vi "CRYDataView Add Panel.vi"(6 "DataView Index":i32, 7 "panel_index":i32, 8 "Selected Panel Idx":i32, 9 "SAdd_Pos":string, 10 "spliter array":refnum<vi>[](array[refnum]), 11 "SubPanel array":refnum<vi>[](array[refnum])) -> (1 "Panel Ref":refnum<vi>, 2 "bResult":bool, 3 "panel_index_out":i32)   [LabVIEW 2013]
uses:
  Control/SplitterBar.ctl
  CRYNew View Global.vi
panel:
  in  "V or H":i32
  in  "cur_position":i32
  in  "parent_spliteridx":i32
  in  "new_add_position":i32
  in  "panel_left":i32
  in  "panel_top":i32
  in  "panel_right":i32
  in  "panel_btm":i32
  in  "cur_panel_top":i32
  in  "cur_panel_left":i32
  in  "cur_panel_hei":i32
  in  "cur_panel_wid":i32
  in  "spliter_index":i32
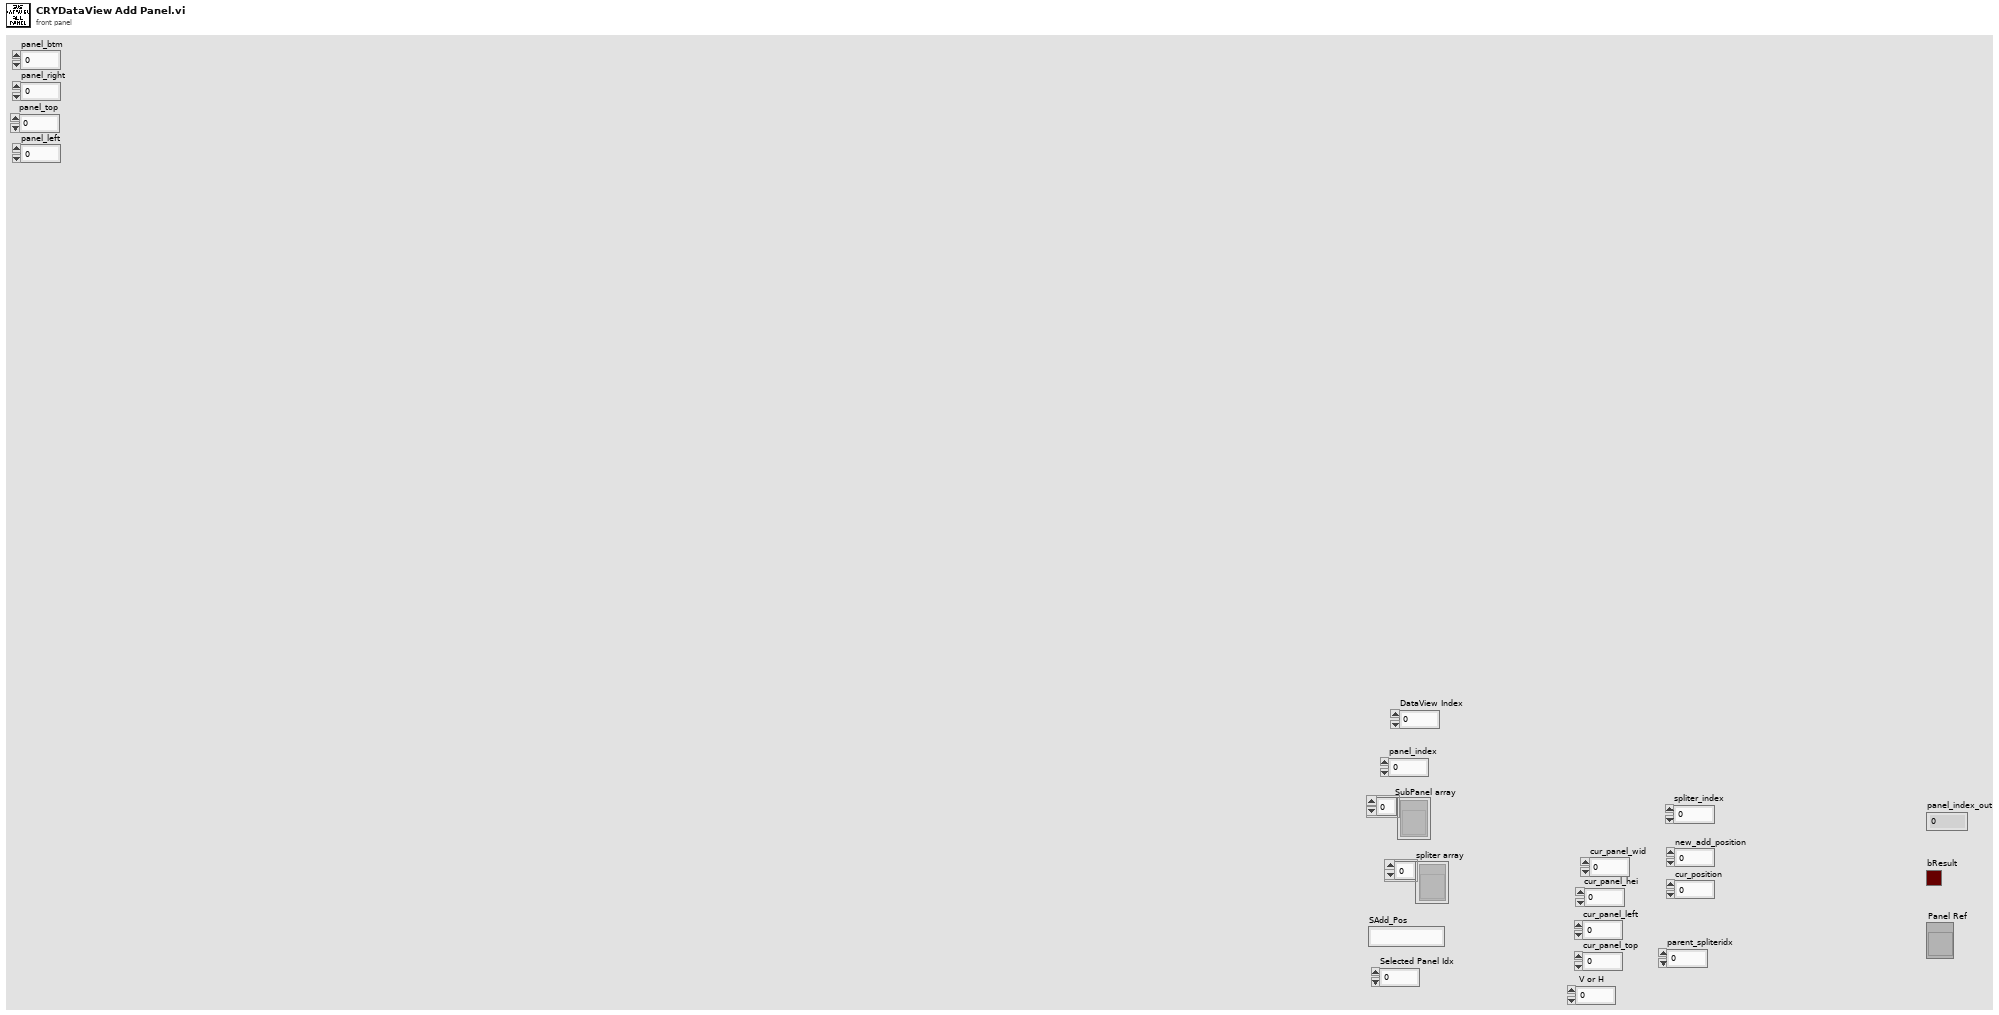
[diagram p1: front panel]
types:
  T1 = typedef "Graph Main Info Cluster.ctl" = cluster{"Selected_BarIdx":i32, "Selected_PanelIdx":i32, "Graph Main VIRef":refnum<vi>, "ToolBarClick":bool, "Spliter Ref Array":refnum<vi>[], "Panel Ref Array":refnum<vi>[], "Spliter_matrix":i32[][], "Panel_matrix":i32[][], "child_spliterIdx_matrix":i32[][], "split_pos_matrix":i32[][], "Title State":bool, "sQueueName":string, "Frame nID":i32, "Graph VIRef Array":cluster{"Graph VIRef":refnum<vi>, "Panel Idx":i32, "Frame VIRef":refnum<vi>, "Icon Ring":i32, "Graph Type":string}[], "View Type":string}
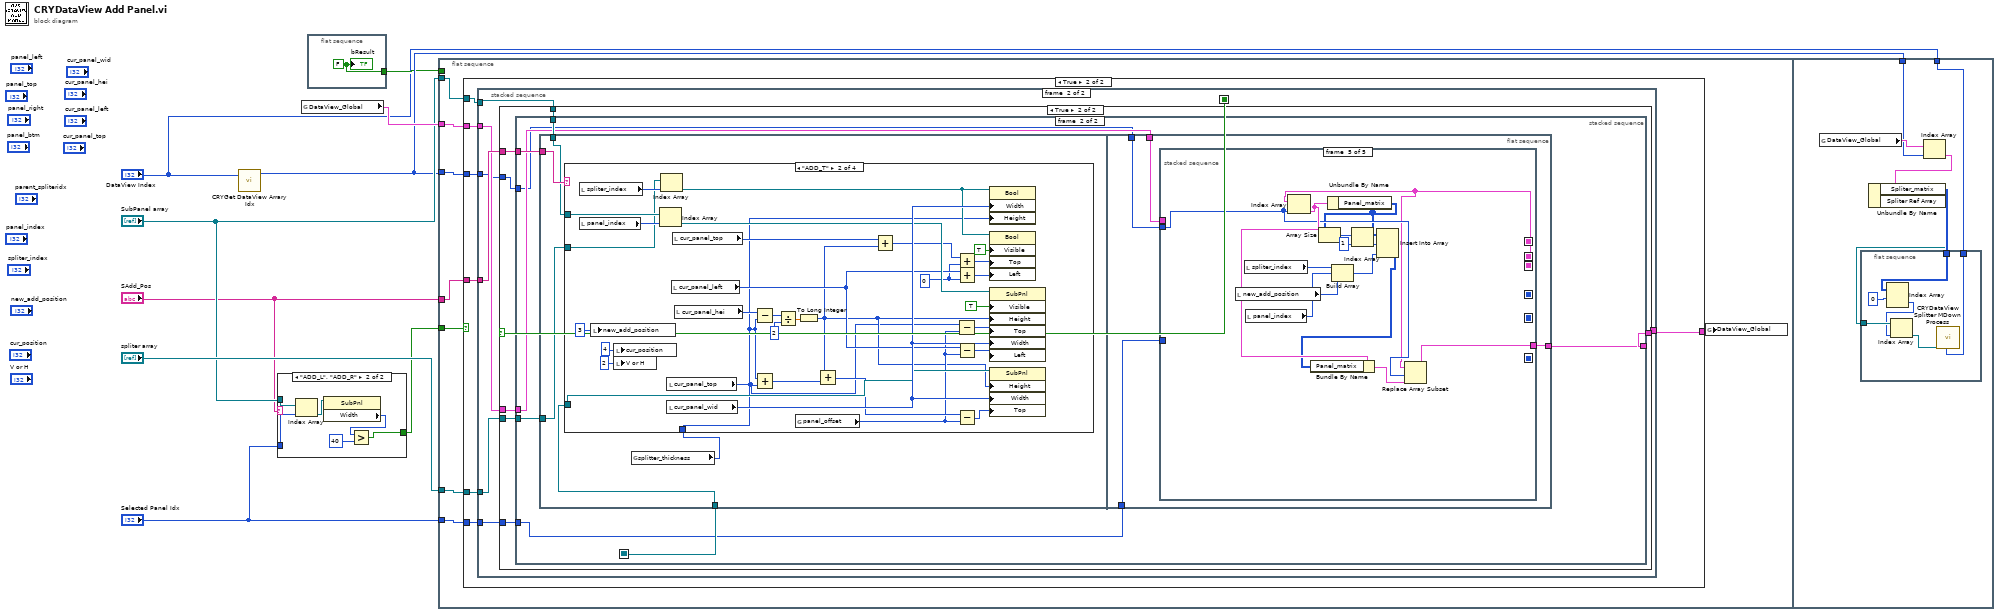
[diagram p0: block diagram]
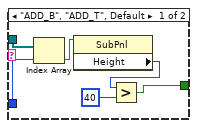
[diagram p2: hidden frame]
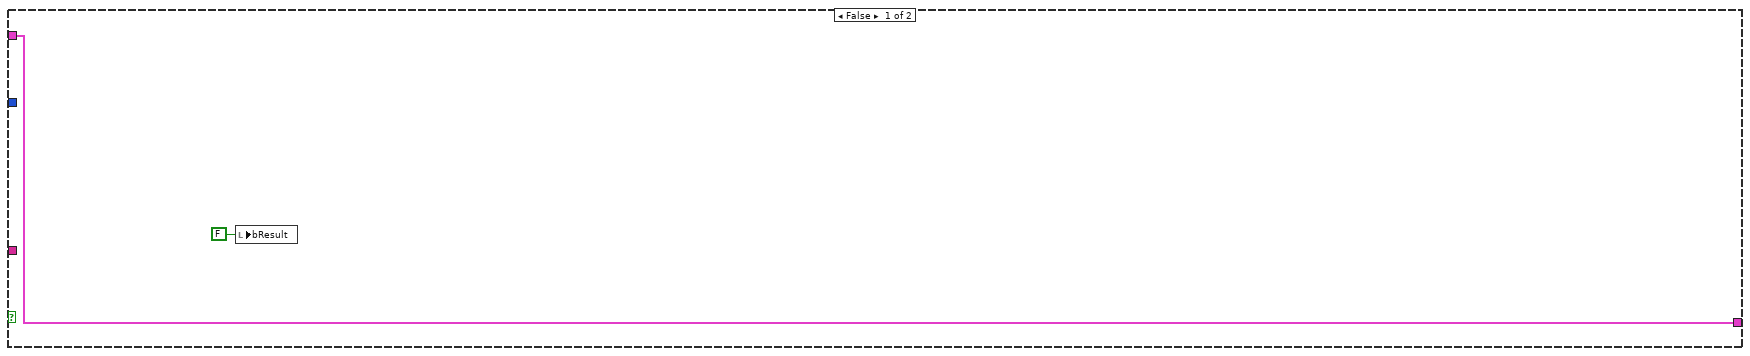
[diagram p3: hidden frame]
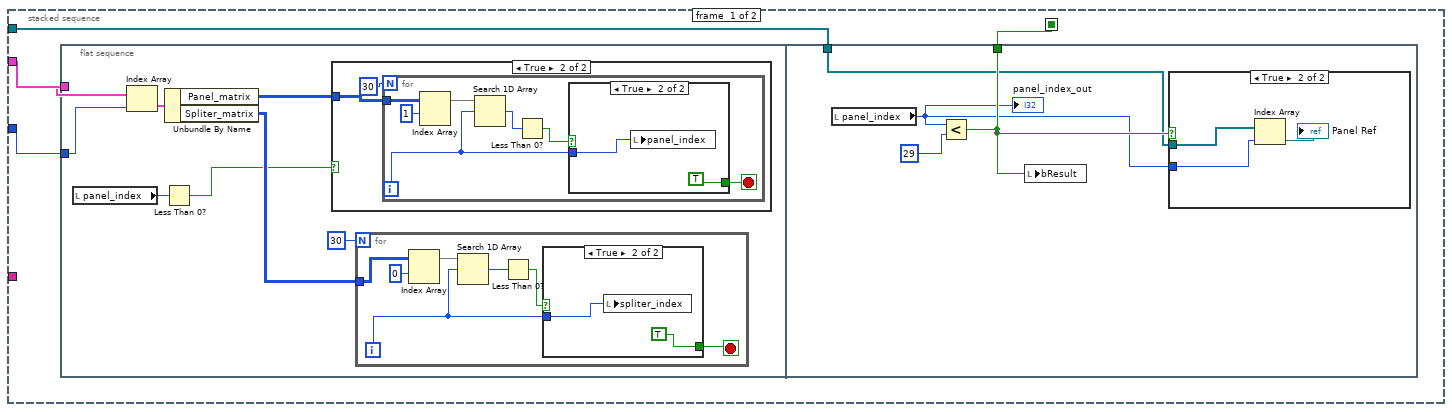
[diagram p4: hidden frame]
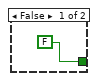
[diagram p6: hidden frame]
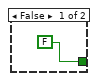
[diagram p7: hidden frame]
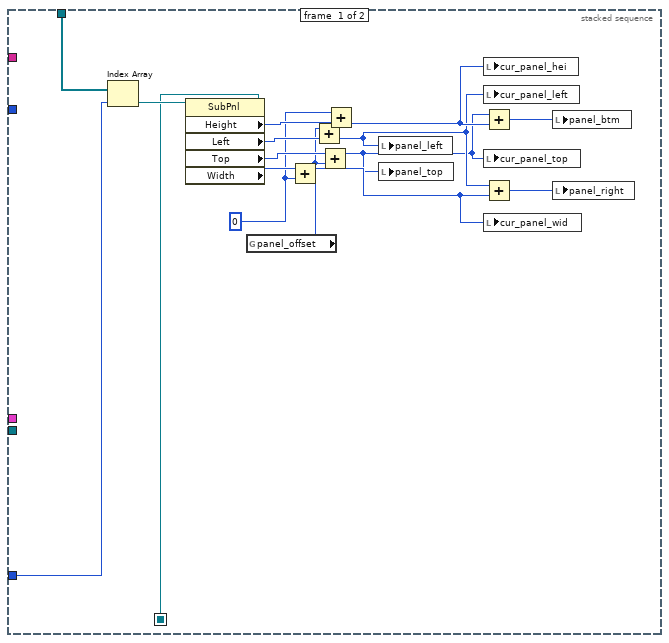
[diagram p10: hidden frame]
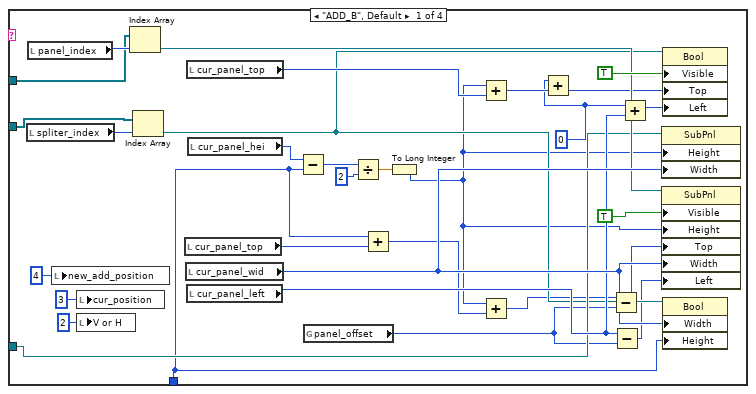
[diagram p11: hidden frame]
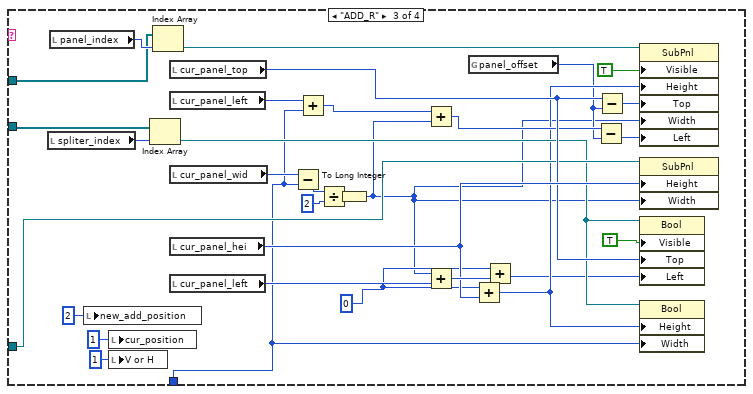
[diagram p12: hidden frame]
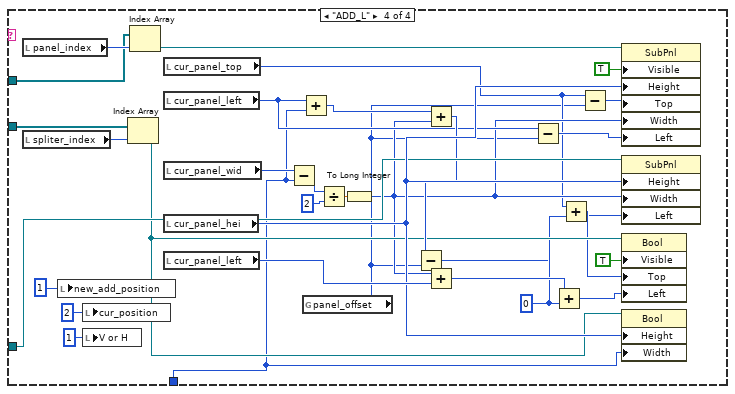
[diagram p13: hidden frame]
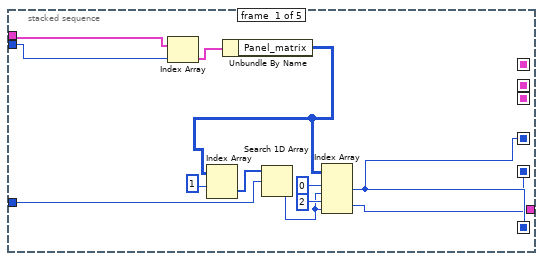
[diagram p14: hidden frame]
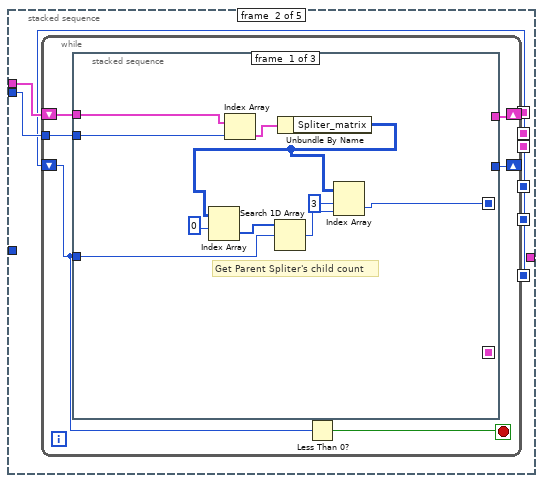
[diagram p15: hidden frame]
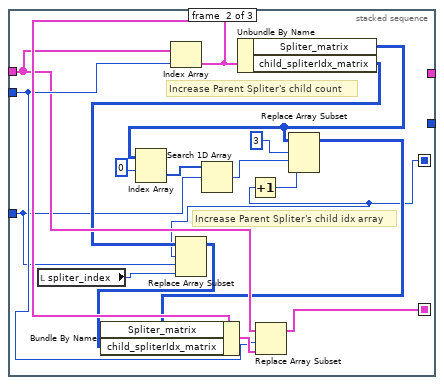
[diagram p16: hidden frame]
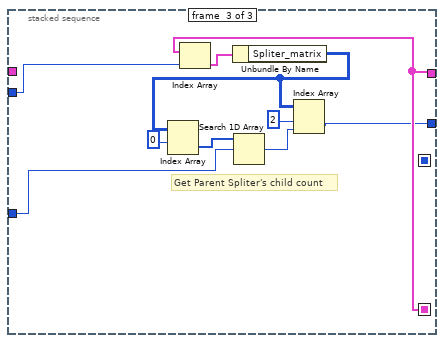
[diagram p17: hidden frame]
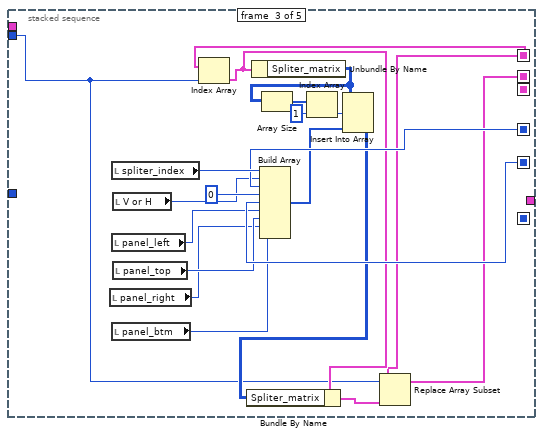
[diagram p18: hidden frame]
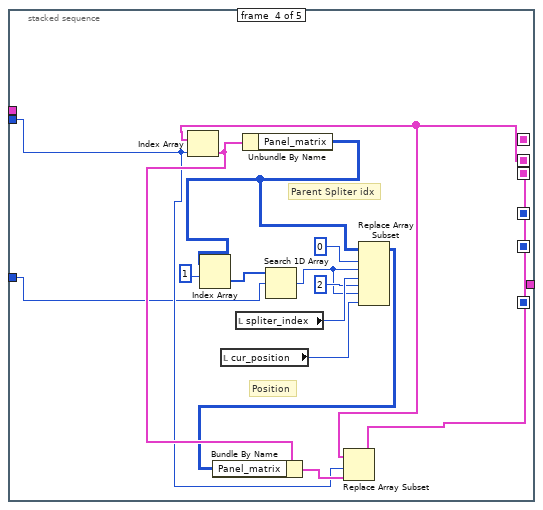
[diagram p19: hidden frame]
diagram:
  n1 = call "CRYGet DataView Arrary Idx.vi"("DataView Idx In"="DataView Index") -> ("DataView Arrary Idx out"=w3:i32)  [unwired: 10 in]
  n2 = case shown="\"ADD_L\", \"ADD_R\"" "SAdd_Pos" {
    tunnel: "Selected Panel Idx" -> [w15 w21]
    tunnel: "SubPanel array" -> [w14 w20]
    tunnel: [w10 w16] -> w4
    frame "ADD_B", "ADD_T", Default {
      n3 = Index Array(array=w14, index=w15) -> (element=w13:refnum<vi>)
      n4 = property class="SubPnl"(reference=w13) -> ("Height"=w12:u32)  [unwired: 1 in, 2 out]
      n5 = Greater?(x=w12, y=u32 40) -> (0:w10:bool)
    }
    frame "ADD_L", "ADD_R" {
      n6 = Index Array(array=w20, index=w21) -> (element=w19:refnum<vi>)
      n7 = property class="SubPnl"(reference=w19) -> ("Width"=w18:u32)  [unwired: 1 in, 2 out]
      n8 = Greater?(x=w18, y=u32 40) -> (0:w16:bool)
    }
  }
  n9 = global read "CRYNew View Global.vi" "DataView_Global"() -> (w9:T1[])
  n10 = flat-sequence {
    tunnel: [w22] -> w2
    frame #0 {
      w22 = FALSE ("bResult")
      "bResult" <- w22
    }
  }
  n11 = flat-sequence {
    tunnel: "SubPanel array" -> [w30]
    tunnel: "spliter array" -> [w29]
    tunnel: "SAdd_Pos" -> [w28]
    tunnel: w9 -> [w27]
    tunnel: w3 -> [w26]
    tunnel: "Selected Panel Idx" -> [w24]
    tunnel: w4 -> [w23]
    tunnel: w2 -> [_]
    tunnel: w3 -> [w365]
    tunnel: "DataView Index" -> [w364]
    frame #0 {
      n12 = case shown="True" w23 {
        tunnel: w30 -> [_ w39]
        tunnel: w29 -> [_ w38]
        tunnel: w28 -> [_ w37]
        tunnel: w27 -> [w32 w36]
        tunnel: w26 -> [_ w35]
        tunnel: [w32 w34] -> w25
        tunnel: w24 -> [_ w33]
        frame False {
          n13 = local write "bResult"(FALSE ("bResult")) -> ()
        }
        frame True {
          n14 = stacked-sequence {
            seq-local: [w40 _] -> [_ w82]
            tunnel: w36 -> [w43 w85]
            tunnel: w35 -> [w42 w84]
            tunnel: w39 -> [w41 w87]
            tunnel: w37 -> [_ w88]
            tunnel: w38 -> [_ w86]
            tunnel: [_ w83] -> w34
            tunnel: w33 -> [_ w81]
            frame #0 {
              n15 = flat-sequence {
                tunnel: w43 -> [w51]
                tunnel: w42 -> [w50]
                tunnel: w41 -> [w75]
                tunnel: [w76] -> w40
                frame #0 {
                  n16 = local read "panel_index"() -> (w49:i32)
                  n17 = Index Array(array=w51, index=w50) -> (element=w47:T1)
                  n18 = Less Than 0?(x=w49) -> (x < 0?=w44:bool)
                  n19 = Unbundle By Name(w47) -> ("Panel_matrix"=w46:i32[][], "Spliter_matrix"=w45:i32[][])
                  n20 = case shown="True" w44 {
                    tunnel: w46 -> [_ w52]
                    frame False {
                    }
                    frame True {
                      n21 = for {
                        N: 30 -> [_]
                        tunnel: w52 -> [w54]
                        i -> [w56]
                        stop <- w55 stop-if-true
                        n22 = Index Array(array=w54, index (row)=1) -> (element=w59:i32[])  [unwired: 1 in]
                        n23 = Search 1D Array(1D array=w59, element=w56) -> (index of element=w58:i32)  [unwired: 1 in]
                        n24 = Less Than 0?(x=w58) -> (x < 0?=w57:bool)
                        n25 = case shown="True" w57 {
                          tunnel: w56 -> [_ w63]
                          tunnel: [FALSE TRUE] -> w55
                          frame False {
                          }
                          frame True {
                            n26 = local write "panel_index"(w63) -> ()
                          }
                        }
                      }
                    }
                  }
                  n27 = for {
                    N: 30 -> [_]
                    tunnel: w45 -> [w64]
                    i -> [w66]
                    stop <- w65 stop-if-true
                    n28 = Index Array(array=w64, index (row)=0) -> (element=w69:i32[])  [unwired: 1 in]
                    n29 = Search 1D Array(1D array=w69, element=w66) -> (index of element=w68:i32)  [unwired: 1 in]
                    n30 = Less Than 0?(x=w68) -> (x < 0?=w67:bool)
                    n31 = case shown="True" w67 {
                      tunnel: w66 -> [_ w73]
                      tunnel: [FALSE TRUE] -> w65
                      frame False {
                      }
                      frame True {
                        n32 = local write "spliter_index"(w73) -> ()
                      }
                    }
                  }
                }
                frame #1 {
                  n33 = local read "panel_index"() -> (w74:i32)
                  "panel_index_out" <- w74
                  n34 = Less?(x=w74, y=29) -> (x < y?=w76:bool)
                  n35 = local write "bResult"(w76) -> ()
                  n36 = case shown="True" w76 {
                    tunnel: w75 -> [_ w80]
                    tunnel: w74 -> [_ w79]
                    frame False {
                    }
                    frame True {
                      n37 = Index Array(array=w80, index=w79) -> (element=→"Panel Ref":refnum<vi>)
                    }
                  }
                }
              }
            }
            frame #1 {
              n38 = case shown="True" w82 {
                tunnel: w88 -> [_ w96]
                tunnel: w87 -> [_ w95]
                tunnel: w86 -> [_ w94]
                tunnel: w85 -> [w89 w93]
                tunnel: w84 -> [_ w92]
                tunnel: [w89 w91] -> w83
                tunnel: w81 -> [_ w90]
                frame False {
                }
                frame True {
                  n39 = stacked-sequence {
                    seq-local: [w104 _] -> [_ w117]
                    tunnel: w96 -> [_ w120]
                    tunnel: w95 -> [w105 w119]
                    tunnel: w94 -> [_ w118]
                    tunnel: w93 -> [_ w116]
                    tunnel: w92 -> [_ w115]
                    tunnel: [_ w114] -> w91
                    tunnel: w90 -> [w103 w113]
                    frame #0 {
                      w100 = 0
                      n40 = Index Array(array=w105, index=w103) -> (element=w106:refnum<vi>)
                      n41 = property class="SubPnl"(reference=w106) -> (reference out=w104:refnum<vi>, "Height"=w111:u32, "Left"=w107:i32, "Top"=w110:i32, "Width"=w109:u32)  [unwired: 1 in, 1 out]
                      n42 = global read "CRYNew View Global.vi" "panel_offset"() -> (w97:i32)
                      n43 = Add(x=w109, y=w100) -> (x+y=w101:u32)
                      n44 = Add(x=w97, y=w107) -> (x+y=w99:i32)
                      n45 = Add(x=w110, y=w97) -> (x+y=w98:i32)
                      n46 = Add(x=w100, y=w111) -> (x+y=w102:u32)
                      n47 = local write "panel_left"(w99) -> ()
                      n48 = local write "panel_top"(w98) -> ()
                      n49 = local write "cur_panel_hei"(w102) -> ()
                      n50 = local write "cur_panel_left"(w99) -> ()
                      n51 = Add(x=w98, y=w102) -> (x+y=w112:u32)
                      n52 = local write "cur_panel_top"(w98) -> ()
                      n53 = Add(x=w99, y=w101) -> (x+y=w108:u32)
                      n54 = local write "cur_panel_wid"(w101) -> ()
                      n55 = local write "panel_btm"(w112) -> ()
                      n56 = local write "panel_right"(w108) -> ()
                    }
                    frame #1 {
                      n57 = flat-sequence {
                        tunnel: w120 -> [w125]
                        tunnel: w119 -> [w124]
                        tunnel: w118 -> [w123]
                        tunnel: w117 -> [w122]
                        tunnel: w116 -> [w255]
                        tunnel: w115 -> [w254]
                        tunnel: [w253] -> w114
                        tunnel: w113 -> [w252]
                        frame #0 {
                          n58 = global read "CRYNew View Global.vi" "splitter_thickness"() -> (w121:u32)
                          n59 = case shown="\"ADD_T\"" w125 {
                            tunnel: w124 -> [w141 w178 w203 w238]
                            tunnel: w123 -> [w140 w177 w202 w237]
                            tunnel: w122 -> [w139 w176 w201 w236]
                            tunnel: w121 -> [w126 w157 w189 w220]
                            frame "ADD_B", Default {
                              w131 = 0
                              n60 = local read "spliter_index"() -> (w156:i32)
                              n61 = local read "panel_index"() -> (w149:i32)
                              n62 = local write "new_add_position"(4 ("new_add_position")) -> ()
                              n63 = local write "cur_position"(3 ("cur_position")) -> ()
                              n64 = local write "V or H"(2 ("V or H")) -> ()
                              n65 = Index Array(array=w141, index=w149) -> (element=w143:refnum<vi>)
                              n66 = Index Array(array=w140, index=w156) -> (element=w135:refnum<vi>)
                              n67 = local read "cur_panel_top"() -> (w147:i32)
                              n68 = local read "cur_panel_wid"() -> (w155:i32)
                              n69 = local read "cur_panel_top"() -> (w151:i32)
                              n70 = local read "cur_panel_left"() -> (w154:i32)
                              n71 = local read "cur_panel_hei"() -> (w146:i32)
                              n72 = Subtract(x=w146, y=w126) -> (x-y=w145:u32)
                              n73 = global read "CRYNew View Global.vi" "panel_offset"() -> (w127:i32)
                              n74 = Divide(x=w145, y=2) -> (x/y=w152:dbl)
                              n75 = Add(x=w126, y=w147) -> (x+y=w148:u32)
                              n76 = To Long Integer(number=w152) -> (32bit integer=w134:i32)
                              n77 = Add(x=w134, y=w151) -> (x+y=w153:i32)
                              n78 = Add(x=w134, y=w148) -> (x+y=w128:u32)
                              n79 = Add(x=w131, y=w153) -> (x+y=w133:i32)
                              n80 = Subtract(x=w128, y=w127) -> (x-y=w129:u32)
                              n81 = Subtract(x=w154, y=w127) -> (x-y=w130:i32)
                              n82 = Add(x=w131, y=w154) -> (x+y=w132:i32)
                              n83 = property class="SubPnl"(reference=w139, "Height"=w134, "Width"=w155) -> ()  [unwired: 1 in, 2 out]
                              n84 = property class="SubPnl"(reference=w143, "Visible"=TRUE, "Height"=w134, "Top"=w129, "Width"=w155, "Left"=w130) -> ()  [unwired: 1 in, 2 out]
                              n85 = property class="Bool"(reference=w135, "Visible"=TRUE, "Top"=w133, "Left"=w132) -> ()  [unwired: 1 in, 2 out]
                              n86 = property class="Bool"(reference=w135, "Width"=w155, "Height"=w126) -> ()  [unwired: 1 in, 2 out]
                            }
                            frame "ADD_T" {
                              w160 = 0
                              n87 = local read "spliter_index"() -> (w188:i32)
                              n88 = local read "panel_index"() -> (w185:i32)
                              n89 = local write "new_add_position"(3 ("new_add_position")) -> ()
                              n90 = local write "cur_position"(4 ("cur_position")) -> ()
                              n91 = local write "V or H"(2 ("V or H")) -> ()
                              n92 = Index Array(array=w178, index=w185) -> (element=w180:refnum<vi>)
                              n93 = Index Array(array=w177, index=w188) -> (element=w171:refnum<vi>)
                              n94 = local read "cur_panel_top"() -> (w158:i32)
                              n95 = local read "cur_panel_wid"() -> (w187:i32)
                              n96 = local read "cur_panel_left"() -> (w165:i32)
                              n97 = local read "cur_panel_top"() -> (w161:i32)
                              n98 = local read "cur_panel_hei"() -> (w183:i32)
                              n99 = Subtract(x=w183, y=w157) -> (x-y=w182:u32)
                              n100 = Add(x=w157, y=w158) -> (x+y=w184:u32)
                              n101 = Divide(x=w182, y=2) -> (x/y=w172:dbl)
                              n102 = global read "CRYNew View Global.vi" "panel_offset"() -> (w163:i32)
                              n103 = To Long Integer(number=w172) -> (32bit integer=w162:i32)
                              n104 = Add(x=w162, y=w184) -> (x+y=w167:u32)
                              n105 = Add(x=w161, y=w162) -> (x+y=w159:i32)
                              n106 = Subtract(x=w158, y=w163) -> (x-y=w164:i32)
                              n107 = Add(x=w159, y=w160) -> (x+y=w170:i32)
                              n108 = Add(x=w165, y=w160) -> (x+y=w169:i32)
                              n109 = Subtract(x=w165, y=w163) -> (x-y=w166:i32)
                              n110 = Subtract(x=w167, y=w163) -> (x-y=w168:u32)
                              n111 = property class="Bool"(reference=w171, "Width"=w187, "Height"=w157) -> ()  [unwired: 1 in, 2 out]
                              n112 = property class="Bool"(reference=w171, "Visible"=TRUE, "Top"=w170, "Left"=w169) -> ()  [unwired: 1 in, 2 out]
                              n113 = property class="SubPnl"(reference=w180, "Visible"=TRUE, "Height"=w162, "Top"=w164, "Width"=w187, "Left"=w166) -> ()  [unwired: 1 in, 2 out]
                              n114 = property class="SubPnl"(reference=w176, "Height"=w162, "Width"=w187, "Top"=w168) -> ()  [unwired: 1 in, 2 out]
                            }
                            frame "ADD_R" {
                              w194 = 0
                              n115 = local read "spliter_index"() -> (w219:i32)
                              n116 = local read "panel_index"() -> (w218:i32)
                              n117 = local write "new_add_position"(2 ("new_add_position")) -> ()
                              n118 = local write "cur_position"(1 ("cur_position")) -> ()
                              n119 = local write "V or H"(1 ("V or H")) -> ()
                              n120 = Index Array(array=w202, index=w219) -> (element=w197:refnum<vi>)
                              n121 = Index Array(array=w203, index=w218) -> (element=w205:refnum<vi>)
                              n122 = local read "cur_panel_top"() -> (w209:i32)
                              n123 = local read "cur_panel_left"() -> (w211:i32)
                              n124 = local read "cur_panel_wid"() -> (w213:i32)
                              n125 = local read "cur_panel_hei"() -> (w214:i32)
                              n126 = local read "cur_panel_left"() -> (w215:i32)
                              n127 = Subtract(x=w213, y=w189) -> (x-y=w210:u32)
                              n128 = Add(x=w211, y=w189) -> (x+y=w212:u32)
                              n129 = Divide(x=w210, y=2) -> (x/y=w216:dbl)
                              n130 = To Long Integer(number=w216) -> (32bit integer=w190:i32)
                              n131 = Add(x=w212, y=w190) -> (x+y=w207:u32)
                              n132 = Add(x=w190, y=w215) -> (x+y=w217:i32)
                              n133 = global read "CRYNew View Global.vi" "panel_offset"() -> (w191:i32)
                              n134 = Add(x=w194, y=w214) -> (x+y=w196:i32)
                              n135 = Add(x=w194, y=w217) -> (x+y=w195:i32)
                              n136 = Subtract(x=w207, y=w191) -> (x-y=w192:u32)
                              n137 = Subtract(x=w209, y=w191) -> (x-y=w193:i32)
                              n138 = property class="SubPnl"(reference=w205, "Visible"=TRUE, "Height"=w196, "Top"=w193, "Width"=w190, "Left"=w192) -> ()  [unwired: 1 in, 2 out]
                              n139 = property class="SubPnl"(reference=w201, "Height"=w214, "Width"=w190) -> ()  [unwired: 1 in, 2 out]
                              n140 = property class="Bool"(reference=w197, "Visible"=TRUE, "Top"=w209, "Left"=w195) -> ()  [unwired: 1 in, 2 out]
                              n141 = property class="Bool"(reference=w197, "Height"=w196, "Width"=w189) -> ()  [unwired: 1 in, 2 out]
                            }
                            frame "ADD_L" {
                              w226 = 0
                              n142 = local read "panel_index"() -> (w250:i32)
                              n143 = local read "spliter_index"() -> (w251:i32)
                              n144 = local write "new_add_position"(1 ("new_add_position")) -> ()
                              n145 = local write "cur_position"(2 ("cur_position")) -> ()
                              n146 = local write "V or H"(1 ("V or H")) -> ()
                              n147 = Index Array(array=w237, index=w251) -> (element=w230:refnum<vi>)
                              n148 = Index Array(array=w238, index=w250) -> (element=w240:refnum<vi>)
                              n149 = local read "cur_panel_top"() -> (w222:i32)
                              n150 = local read "cur_panel_left"() -> (w234:i32)
                              n151 = local read "cur_panel_wid"() -> (w245:i32)
                              n152 = local read "cur_panel_hei"() -> (w246:i32)
                              n153 = local read "cur_panel_left"() -> (w247:i32)
                              n154 = Subtract(x=w245, y=w220) -> (x-y=w243:u32)
                              n155 = Add(x=w234, y=w220) -> (x+y=w244:u32)
                              n156 = global read "CRYNew View Global.vi" "panel_offset"() -> (w221:i32)
                              n157 = Divide(x=w243, y=2) -> (x/y=w248:dbl)
                              n158 = To Long Integer(number=w248) -> (32bit integer=w229:i32)
                              n159 = Add(x=w244, y=w229) -> (x+y=w235:u32)
                              n160 = Subtract(x=w235, y=w221) -> (x-y=w225:u32)
                              n161 = Add(x=w229, y=w247) -> (x+y=w249:i32)
                              n162 = Subtract(x=w234, y=w221) -> (x-y=w224:i32)
                              n163 = Add(x=w249, y=w226) -> (x+y=w228:i32)
                              n164 = Add(x=w222, y=w226) -> (x+y=w227:i32)
                              n165 = Subtract(x=w222, y=w221) -> (x-y=w223:i32)
                              n166 = property class="SubPnl"(reference=w240, "Visible"=TRUE, "Height"=w246, "Top"=w223, "Width"=w229, "Left"=w224) -> ()  [unwired: 1 in, 2 out]
                              n167 = property class="SubPnl"(reference=w236, "Height"=w246, "Width"=w229, "Left"=w225) -> ()  [unwired: 1 in, 2 out]
                              n168 = property class="Bool"(reference=w230, "Visible"=TRUE, "Top"=w227, "Left"=w228) -> ()  [unwired: 1 in, 2 out]
                              n169 = property class="Bool"(reference=w230, "Height"=w246, "Width"=w220) -> ()  [unwired: 1 in, 2 out]
                            }
                          }
                        }
                        frame #1 {
                          n170 = stacked-sequence {
                            seq-local: [w258 _ _ _ _] -> [_ _ w332 _ _]
                            seq-local: [w257 _ _ _ _] -> [_ _ w331 _ _]
                            seq-local: [w258 _ _ _ _] -> [_ w269 _ _ _]
                            seq-local: [_ w268 _ _ _] -> [_ _ w325 _ _]
                            seq-local: [_ _ w324 _ _] -> [_ _ _ w344 _]
                            seq-local: [_ _ _ w343 _] -> [_ _ _ _ w358]
                            tunnel: w255 -> [w264 w271 _ _ _]
                            tunnel: w254 -> [w263 w270 w315 w345 w359]
                            tunnel: [_ _ _ _ w357] -> w253
                            tunnel: w252 -> [w262 _ _ w342 _]
                            frame #0 {
                              n171 = Index Array(array=w264, index=w263) -> (element=w265:T1)
                              n172 = Unbundle By Name(w265) -> ("Panel_matrix"=w256:i32[][])
                              n173 = Index Array(array=w256, index (row)=1 ("row 1")) -> (element=w267:i32[])  [unwired: 1 in]
                              n174 = Search 1D Array(1D array=w267, element=w262) -> (index of element=w259:i32)  [unwired: 1 in]
                              n175 = Index Array(array=w256, index (row) #1=0 ("index (row)"), index (col) #1=w259, index (row) #2=2 ("index (row)"), index (col) #2=w259) -> (element #1=w258:i32, element #2=w257:i32)
                            }
                            frame #1 {
                              n176 = while {
                                shift-right: [w277] -> _
                                shift-left: w269 -> [w276]
                                tunnel: w270 -> [w273]
                                shift-right: [w272] -> w268
                                shift-left: w271 -> [w274]
                                stop <- w275 stop-if-true
                                n177 = stacked-sequence {
                                seq-local: [w279 _ _] -> [_ w292 _]
                                seq-local: [_ w298 _] -> [_ _ w309]
                                tunnel: w276 -> [w285 w291 w312]
                                tunnel: [_ _ w306] -> w277
                                tunnel: w274 -> [w283 w299 _]
                                tunnel: w273 -> [w282 w300 w310]
                                tunnel: [_ _ w309] -> w272
                                frame #0 {
                                # "Get Parent Spliter's child count"
                                n178 = Index Array(array=w283, index=w282) -> (element=w284:T1)
                                n179 = Unbundle By Name(w284) -> ("Spliter_matrix"=w278:i32[][])
                                n180 = Index Array(array=w278, index (row)=0 ("row 1")) -> (element=w286:i32[])  [unwired: 1 in]
                                n181 = Search 1D Array(1D array=w286, element=w285) -> (index of element=w280:i32)  [unwired: 1 in]
                                n182 = Index Array(array=w278, index (row)=3, index (col)=w280) -> (element=w279:i32)
                                }
                                frame #1 {
                                # "Increase Parent Spliter's child idx array"
                                # "Increase Parent Spliter's child count"
                                n183 = local read "spliter_index"() -> (w290:i32)
                                n184 = Index Array(array=w299, index=w300) -> (element=w301:T1)
                                n185 = Unbundle By Name(w301) -> ("Spliter_matrix"=w288:i32[][], "child_spliterIdx_matrix"=w293:i32[][])
                                n186 = Index Array(array=w288, index (row)=0 ("row 1")) -> (element=w303:i32[])  [unwired: 1 in]
                                n187 = Replace Array Subset(array=w293, new element=w290, index (row)=w292, index (col)=w291) -> (w289:i32[][])
                                n188 = Search 1D Array(1D array=w303, element=w291) -> (index of element=w296:i32)  [unwired: 1 in]
                                n189 = Increment(x=w292) -> (x+1=w297:i32)
                                n190 = Replace Array Subset(array=w288, new element=w297, index (row)=3 ("disabled index (row)"), index (col)=w296) -> (w294:i32[][])
                                n191 = Bundle By Name(cluster=w301, "Spliter_matrix"=w294, "child_spliterIdx_matrix"=w289) -> (w302:T1)
                                n192 = Replace Array Subset(array=w299, new element=w302, index=w300) -> (w298:T1[])
                                }
                                frame #2 {
                                # "Get Parent Spliter's child count"
                                n193 = Index Array(array=w309, index=w310) -> (element=w311:T1)
                                n194 = Unbundle By Name(w311) -> ("Spliter_matrix"=w305:i32[][])
                                n195 = Index Array(array=w305, index (row)=0 ("row 1")) -> (element=w313:i32[])  [unwired: 1 in]
                                n196 = Search 1D Array(1D array=w313, element=w312) -> (index of element=w307:i32)  [unwired: 1 in]
                                n197 = Index Array(array=w305, index (row)=2, index (col)=w307) -> (element=w306:i32)
                                }
                                }
                                n198 = Less Than 0?(x=w276) -> (x < 0?=w275:bool)
                              }
                            }
                            frame #2 {
                              n199 = local read "panel_right"() -> (w329:i32)
                              n200 = local read "spliter_index"() -> (w333:i32)
                              n201 = local read "panel_left"() -> (w323:i32)
                              n202 = local read "panel_btm"() -> (w328:i32)
                              n203 = local read "V or H"() -> (w322:i32)
                              n204 = local read "panel_top"() -> (w330:i32)
                              n205 = Index Array(array=w325, index=w315) -> (element=w326:T1)
                              n206 = Unbundle By Name(w326) -> ("Spliter_matrix"=w319:i32[][])
                              n207 = Build Array(w333, w322, w332, 0 ("element"), w331, w323, w330, w329, w328) -> (w317:i32[])
                              n208 = Array Size(array=w319) -> (size(s)=w321:i32[])
                              n209 = Index Array(array=w321, index=1) -> (element=w318:i32)
                              n210 = Insert Into Array(array=w319, index (col)=w318, new element=w317) -> (w316:i32[][])  [unwired: 1 in]
                              n211 = Bundle By Name(cluster=w326, "Spliter_matrix"=w316) -> (w327:T1)
                              n212 = Replace Array Subset(array=w325, new element=w327, index=w315) -> (w324:T1[])
                            }
                            frame #3 {
                              # "Position"
                              # "Parent Spliter idx"
                              n213 = Index Array(array=w344, index=w345) -> (element=w346:T1)
                              n214 = local read "cur_position"() -> (w336:i32)
                              n215 = local read "spliter_index"() -> (w339:i32)
                              n216 = Unbundle By Name(w346) -> ("Panel_matrix"=w341:i32[][])
                              n217 = Index Array(array=w341, index (row)=1 ("row 1")) -> (element=w348:i32[])  [unwired: 1 in]
                              n218 = Search 1D Array(1D array=w348, element=w342) -> (index of element=w337:i32)  [unwired: 1 in]
                              n219 = Replace Array Subset(array=w341, new element #1=w339, index (row) #1=0 ("disabled index (row)"), index (col) #1=w337, new element #2=w336, index (row) #2=2 ("disabled index (row)"), index (col) #2=w337) -> (w335:i32[][])
                              n220 = Bundle By Name(cluster=w346, "Panel_matrix"=w335) -> (w347:T1)
                              n221 = Replace Array Subset(array=w344, new element=w347, index=w345) -> (w343:T1[])
                            }
                            frame #4 {
                              n222 = local read "new_add_position"() -> (w356:i32)
                              n223 = local read "spliter_index"() -> (w362:i32)
                              n224 = local read "panel_index"() -> (w363:i32)
                              n225 = Index Array(array=w358, index=w359) -> (element=w360:T1)
                              n226 = Unbundle By Name(w360) -> ("Panel_matrix"=w352:i32[][])
                              n227 = Array Size(array=w352) -> (size(s)=w355:i32[])
                              n228 = Build Array(w362, w363, w356) -> (w350:i32[])
                              n229 = Index Array(array=w355, index=1) -> (element=w353:i32)
                              n230 = Insert Into Array(array=w352, index (col)=w353, new element=w350) -> (w351:i32[][])  [unwired: 1 in]
                              n231 = Bundle By Name(cluster=w360, "Panel_matrix"=w351) -> (w361:T1)
                              n232 = Replace Array Subset(array=w358, new element=w361, index=w359) -> (w357:T1[])
                            }
                          }
                        }
                      }
                    }
                  }
                }
              }
            }
          }
        }
      }
      n233 = global write "CRYNew View Global.vi" "DataView_Global"(w25) -> ()
    }
    frame #1 {
      n234 = global read "CRYNew View Global.vi" "DataView_Global"() -> (w369:T1[])
      n235 = flat-sequence {
        tunnel: w366 -> [w375]
        tunnel: w367 -> [w373]
        tunnel: w364 -> [w370]
        frame #0 {
          w372 = 0 ("index (row)")
          n236 = Index Array(array=w373, index (row)=w372, index (col)=w372) -> (element=w371:i32)
          n237 = Index Array(array=w375, index=w371) -> (element=w374:refnum<vi>)
          n238 = call "CRYDataView Splitter MDown Process.vi"("DataView Index"=w370, "Selected Spliter Ref"=w374) -> ()  [unwired: 9 in, 1 out]
        }
      }
      n239 = Index Array(array=w369, index=w365) -> (element=w368:T1)
      n240 = Unbundle By Name(w368) -> ("Spliter_matrix"=w367:i32[][], "Spliter Ref Array"=w366:refnum<vi>[])
    }
  }
